vi "orderbook.test.Order.Executed.Partialvi.vi"(8 "error in":errorcluster) -> (0 "error out":errorcluster, 3 "Passed":bool)   [LabVIEW 2020]
uses:
  arty/orderbook/orderbook.command.ctl
  arty/orderbook/orderbook.command.type.ctl
  arty/application/orderbook.entry.ctl
  arty/application/orderbook.result.type.ctl
panel:
  out "Counters":T1
  out "OrderBook.Entries":T2[](array[typedef]) {"Side (U8)" format="%.0x"; "Order Id (U64)" format="%.0x"}
  in  "OrderBook.Command[]\nto Send":T4[](array[typedef])=[{"OrderBook Command.Type"=enum."AddOrder", "Side (U8)"=66, "Order Id (U64)"=4617, "Quantity (U32)"=130, "Symbol (U64)"=29033, "Price (U64)"=9525, "Executed Quantity (U32)"=0, "Cancelled Quantity (U32)"=0}, {"OrderBook Command.Type"=enum."AddOrder", "Side (U8)"=66, "Order Id (U64)"=4618, "Quantity (U32)"=225, "Symbol (U64)"=29033, "Price (U64)"=9115, "Executed Quantity (U32)"=0, "Cancelled Quantity (U32)"=0}, {"OrderBook Command.Type"=enum."OrderExecuted", "Side (U8)"=0, "Order Id (U64)"=4617, "Quantity (U32)"=0, "Symbol (U64)"=0, "Price (U64)"=0, "Executed Quantity (U32)"=100, "Cancelled Quantity (U32)"=0}, {"OrderBook Command.Type"=enum."Get.All.Orders", "Side (U8)"=66, "Order Id (U64)"=0, "Quantity (U32)"=0, "Symbol (U64)"=0, "Price (U64)"=0, "Executed Quantity (U32)"=0, "Cancelled Quantity (U32)"=0}] {"Side (U8)" format="%.0x"; "Order Id (U64)" format="%.0x"; "Symbol (U64)" format="%.0x"}
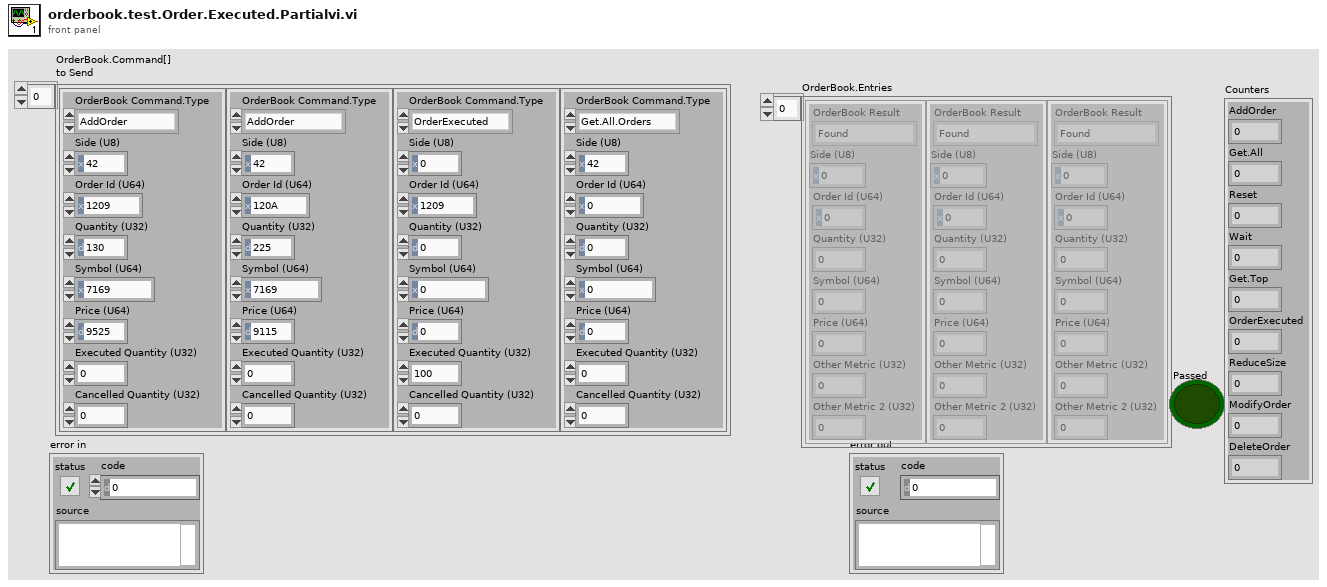
[diagram p1: front panel]
types:
  T1 = cluster{"AddOrder":u32, "Get.All":u32, "Reset":u32, "Wait":u32, "Get.Top":u32, "OrderExecuted":u32, "ReduceSize":u32, "ModifyOrder":u32, "DeleteOrder":u32}
  T2 = typedef "orderbook.entry.ctl" = cluster{"OrderBook Result":T3, "Side (U8)":u8, "Order Id (U64)":u64, "Quantity (U32)":u32, "Symbol (U64)":u64, "Price (U64)":u64, "Other Metric (U32)":u32, "Other Metric 2 (U32)":u32}
  T3 = typedef "orderbook.result.type.ctl" = enum16{"Found", "Not.Found"}
  T4 = typedef "orderbook.command.ctl" = cluster{"OrderBook Command.Type":T5, "Side (U8)":u8, "Order Id (U64)":u64, "Quantity (U32)":u32, "Symbol (U64)":u64, "Price (U64)":u64, "Executed Quantity (U32)":u32, "Cancelled Quantity (U32)":u32}
  T5 = typedef "orderbook.command.type.ctl" = enum16{"AddOrder", "OrderExecuted", "ReduceSize", "ModifyOrder", "DeleteOrder", "Get.All.Orders", "Get.Top"}
  T6 = cluster{"Write.Request":bool, "Read.Request":bool, "Read.Address":u32, "Read.OrderBook.Entry":cluster{"OrderBook Result":enum16{"Found", "Not.Found"}, "Side (U8)":u8, "Order Id (U64)":u64, "Quantity (U32)":u32, "Symbol (U64)":u64, "Price (U64)":u64, "Other Metric (U32)":u32, "Other Metric 2 (U32)":u32}, "Number.of.Entries":u32, "OrderBook.State":enum16{"Reset", "Wait", "Get.Top", "Get.All.Orders", "AddOrder", "Order.Executed", "Reduce.Size", "Modify.Order", "Delete.Order"}, "Ready.For.OrderBook.Command":bool, "Memory.State":enum16{"New", "Request.Data", "Append", "Data.Ready"}, "Move":bool, "Read.Valid":bool, "Write.Address":u32, "Write.OrderBook.Entry":cluster{"OrderBook Result":enum16{"Found", "Not.Found"}, "Side (U8)":u8, "Order Id (U64)":u64, "Quantity (U32)":u32, "Symbol (U64)":u64, "Price (U64)":u64, "Other Metric (U32)":u32, "Other Metric 2 (U32)":u32}, "OrderBook.Result.Valid":bool, "Append":bool, "Counters":cluster{"AddOrder":u32, "Get.All":u32, "Reset":u32, "Wait":u32, "Get.Top":u32, "OrderExecuted":u32, "ReduceSize":u32, "ModifyOrder":u32, "DeleteOrder":u32}}
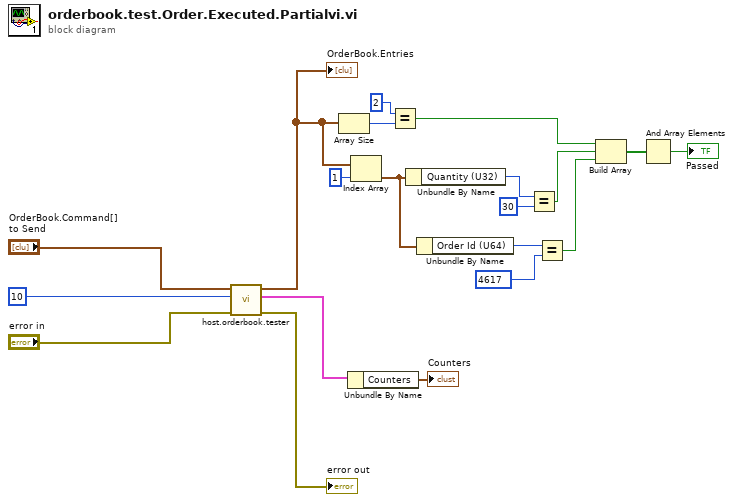
[diagram p0: block diagram]
diagram:
  n1 = call "host.orderbook.tester.vi"("error in"="error in", "Seconds to Wait"=10 ("Seconds\nto\nWait"), "OrderBook.Command[]\nto Send"="OrderBook.Command[]\nto Send") -> ("error out"=→"error out":errorcluster, "OrderBook.Variables"=w2:T6, "OrderBook.Entries"=w8:T2[])  [unwired: 6 in]
  "OrderBook.Entries" <- w8
  n2 = Array Size(array=w8) -> (size(s)=w17:i32)
  n3 = Unbundle By Name(w2) -> ("Counters"=→"Counters":T1)
  n4 = Index Array(array=w8, index=1) -> (element=w7:T2)
  n5 = Equal?(x=2, y=w17) -> (x = y?=w12:bool)
  n6 = Unbundle By Name(w7) -> ("Quantity (U32)"=w14:u32)
  n7 = Unbundle By Name(w7) -> ("Order Id (U64)"=w6:u64)
  n8 = Equal?(x=w14, y=u32 30) -> (x = y?=w13:bool)
  n9 = Equal?(x=w6, y=u64 4617) -> (x = y?=w5:bool)
  n10 = Build Array(w12, w13, w5) -> (w11:bool[])
  n11 = And Array Elements(Boolean array=w11) -> (logical AND=→"Passed":bool)
